vi "Run.vi"(7 "Team Index":i32, 8 "Column":i32, 9 "Row":i32, 10 "View":i32[](array[numeric]) caption="View (Team Index, -1: empty)", 11 "Runner in":refnum<class "Pinwheel.lvclass">) -> (0 "Replicated":refnum<class "Square.lvclass">, 1 "Direction":T1, 2 "Action":T2, 3 "Square Out":refnum<class "Square.lvclass">)   [LabVIEW 2015, in "Pinwheel.lvclass"]
uses:
  Pinwheel.lvclass
  Square/Square.lvclass
  Type Defs/Action Enum.ctl
  Type Defs/Direction Enum.ctl
  DVR Cluster.ctl
  Pinwheel.lvclass/Pinwheel.ctl
  SubVIs/Read-Only Globals.vi
  SubVIs/Globals (private).vi
  Type Defs/SB Type Defs.lvlib
panel:
  # "NW\nN\nNE\nE\nSE\nS\nSW\nW"
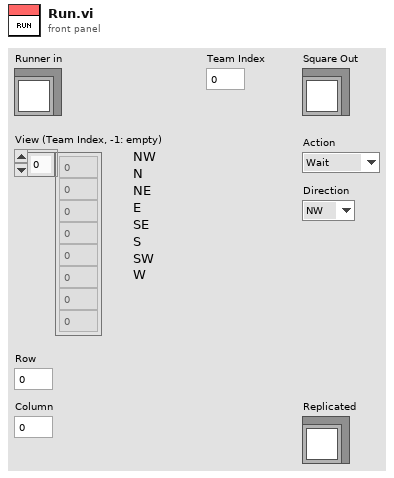
[diagram p1: front panel]
types:
  T1 = typedef "SB Type Defs.lvlib/Direction Enum.ctl" = enum16{"NW", "N", "NE", "E", "SE", "S", "SW", "W"}
  T2 = typedef "SB Type Defs.lvlib/Action Enum.ctl" = enum16{"Wait", "Move", "Attack", "Replicate"}
  T3 = typedef "Pinwheel.lvclass/DVR Cluster.ctl" = cluster{"N":i32, "E":i32, "S":i32, "W":i32, "OD":T1, "NR":i32, "ER":i32, "SR":i32, "WR":i32, "NE":i32, "EE":i32, "SE":i32, "WE":i32, "Team":i32}
  T4 = typedef "Pinwheel.lvclass/Ring Enum.ctl" = enum16{"Defense", "Fill", "Outer", "Inner"}
  T5 = typedef "Pinwheel.lvclass/Role Enum.ctl" = enum16{"Parent", "Move", "Child"}
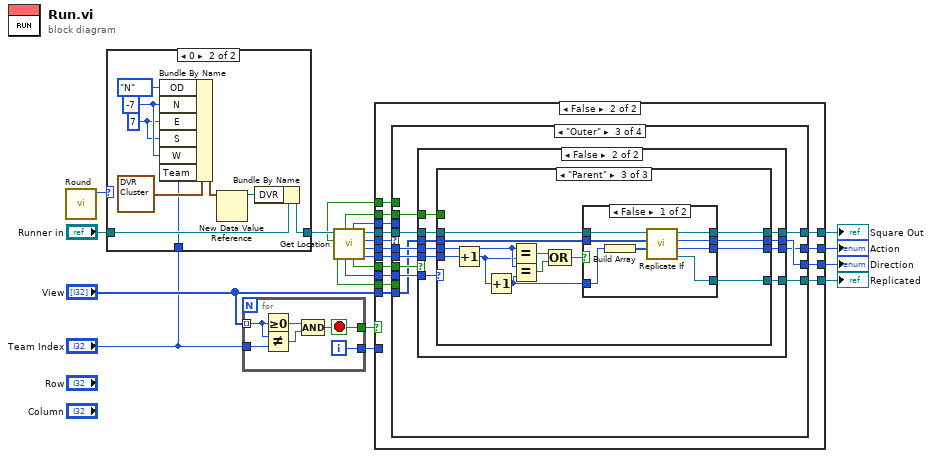
[diagram p0: block diagram]
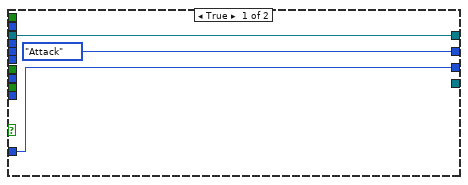
[diagram p2: hidden frame]
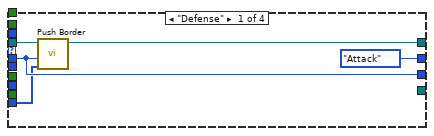
[diagram p3: hidden frame]
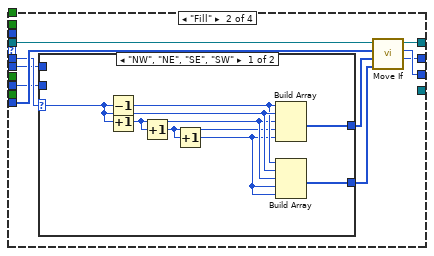
[diagram p4: hidden frame]
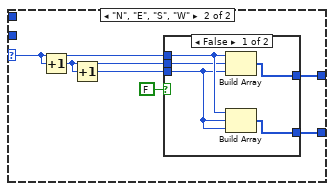
[diagram p5: hidden frame]
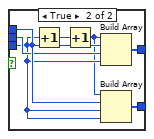
[diagram p6: hidden frame]
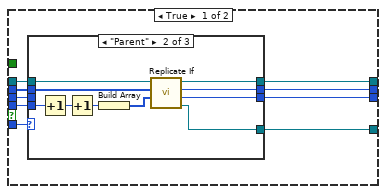
[diagram p7: hidden frame]
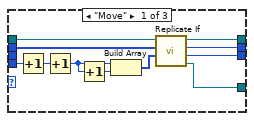
[diagram p8: hidden frame]
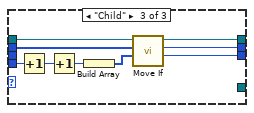
[diagram p9: hidden frame]
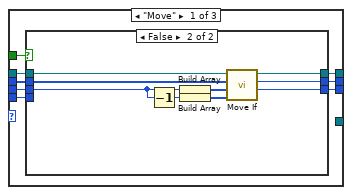
[diagram p10: hidden frame]
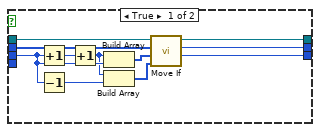
[diagram p11: hidden frame]
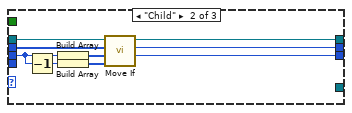
[diagram p12: hidden frame]
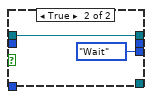
[diagram p13: hidden frame]
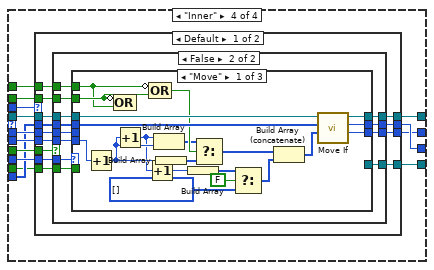
[diagram p14: hidden frame]
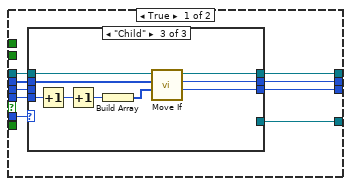
[diagram p15: hidden frame]
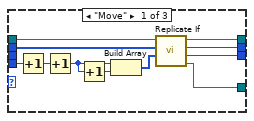
[diagram p16: hidden frame]
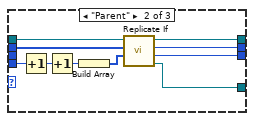
[diagram p17: hidden frame]
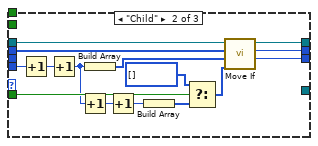
[diagram p18: hidden frame]
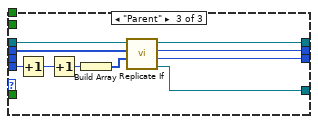
[diagram p19: hidden frame]
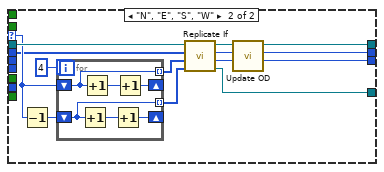
[diagram p20: hidden frame]
diagram:
  n1 = call "Round.vi"() -> ("Round"=w21:i32)  [unwired: 11 in]
  n2 = case shown="0" w21 {
    tunnel: "Runner in" -> [w22 w31]
    tunnel: [w22 w29] -> w19
    tunnel: "Team Index" -> [_ w23]
    frame Default {
    }
    frame 0 {
      w25 = 7 ("E")
      w26 = -7 ("N")
      n3 = Bundle By Name(cluster=T3 {"N"=0, "E"=0, "S"=0, "W"=0, "OD"=enum."NW", "NR"=0, "ER"=0, "SR"=0, "WR"=0, "NE"=0, "EE"=0, "SE"=0, "WE"=0, "Team"=0} ("DVR Cluster"), "OD"=Direction_Enum."N", "N"=w26, "E"=w25, "S"=w25, "W"=w26, "Team"=w23) -> (w27:T3)
      n4 = New Data Value Reference(data value=w27) -> (data value reference=w30:refnum<data-value>)  [unwired: 1 in, 1 out]
      n5 = Bundle By Name(cluster=w31, "DVR"=w30) -> (w29:refnum<class "Pinwheel.lvclass">)
    }
  }
  n6 = for {
    tunnel: "View" -> [w35] mode=indexing
    tunnel: "Team Index" -> [w36]
    tunnel: [w33] -> w3
    tunnel: [w32] -> w2
    i -> [w33]
    stop <- w32 stop-if-true
    n7 = Greater Or Equal To 0?(x=w35) -> (x >= 0?=w37:bool)
    n8 = Not Equal?(x=w35, y=w36) -> (x != y?=w34:bool)
    n9 = Compound Arithmetic op=AND(w37, w34) -> (w32:bool)
  }
  n10 = call "Get Location.vi"("Class"=w19) -> ("Clan"=w11:T1, "Post"=w12:T1, "Ring"=w13:T4, "Class"=w14:refnum<class "Pinwheel.lvclass">, "Diagonal"=w10:bool, "OD"=w8:T1, "Role"=w9:T5, "Jump"=w7:bool, "Move Anyway"=w6:bool, "Chute"=w5:bool)  [unwired: 1 in]
  n11 = case shown="False" w2 {
    tunnel: w14 -> [w40 w55]
    tunnel: [w40 w54] -> w18
    tunnel: [w38 w53] -> w17
    tunnel: [Action_Enum."Attack" ("Action") w52] -> w16
    tunnel: [_ w51] -> w15
    tunnel: "View" -> [_ w50]
    tunnel: w13 -> [_ w49]
    tunnel: w12 -> [_ w48]
    tunnel: w11 -> [_ w47]
    tunnel: w10 -> [_ w46]
    tunnel: w9 -> [_ w45]
    tunnel: w8 -> [_ w44]
    tunnel: w7 -> [_ w43]
    tunnel: w6 -> [_ w42]
    tunnel: w5 -> [_ w41]
    tunnel: w3 -> [w38 _]
    frame True {
    }
    frame False {
      n12 = case shown="\"Outer\"" w49 {
        tunnel: [w58 w69 w101 w224] -> w54
        tunnel: w55 -> [w59 w70 w102 w225]
        tunnel: w48 -> [w57 w65 w104 w227]
        tunnel: w50 -> [w56 w68 w98 w221]
        tunnel: [w57 w67 w100 w223] -> w53
        tunnel: [Action_Enum."Attack" ("Action") w66 w99 w222] -> w52
        tunnel: [_ _ w97 w220] -> w51
        tunnel: w47 -> [_ w61 w103 w226]
        tunnel: w46 -> [_ _ w106 w229]
        tunnel: w45 -> [_ w62 w105 w228]
        tunnel: w44 -> [_ _ _ w219]
        tunnel: w43 -> [_ _ w96 w218]
        tunnel: w42 -> [_ _ _ w217]
        tunnel: w41 -> [_ _ _ w216]
        frame "Defense" {
          n13 = call "Push Border.vi"("1D Maze"=w56, "Post"=w57, "Class"=w59) -> ("Class"=w58:refnum<class "Pinwheel.lvclass">)  [unwired: 8 in]
        }
        frame "Fill" {
          n14 = case shown="\"NW\", \"NE\", \"SE\", \"SW\"" w65 {
            selector: w65 -> [w77 w83]
            tunnel: [w76 w82] -> w64
            tunnel: [w75 w81] -> w63
            tunnel: w62 -> [_ _]
            tunnel: w61 -> [_ _]
            frame "NW", "NE", "SE", "SW" {
              n15 = Decrement(x=w77) -> (x-1=w74:T1)
              n16 = Increment(x=w77) -> (x+1=w73:T1)
              n17 = Increment(x=w73) -> (x+1=w72:T1)
              n18 = Increment(x=w72) -> (x+1=w71:T1)
              n19 = Build Array(w74, w77, w73, w72, w71) -> (w76:T1[])
              n20 = Build Array(w74, w77, w73, w71, w71) -> (w75:T1[])
            }
            frame "N", "E", "S", "W" {
              n21 = Increment(x=w83) -> (x+1=w80:T1)
              n22 = Increment(x=w80) -> (x+1=w79:T1)
              n23 = case shown="False" FALSE {
                tunnel: [w88 w95] -> w82
                tunnel: w83 -> [w87 w94]
                tunnel: w80 -> [w86 w93]
                tunnel: [w85 w92] -> w81
                tunnel: w79 -> [w84 w91]
                frame False {
                  n24 = Build Array(w87, w86, w84) -> (w88:T1[])
                  n25 = Build Array(w87, w84, w84) -> (w85:T1[])
                }
                frame True {
                  n26 = Increment(x=w91) -> (x+1=w90:T1)
                  n27 = Increment(x=w90) -> (x+1=w89:T1)
                  n28 = Build Array(w89, w94, w93, w91) -> (w95:T1[])
                  n29 = Build Array(w89, w94, w91, w91) -> (w92:T1[])
                }
              }
            }
          }
          n30 = call "Move If.vi"("If"=w63, "Move"=w64, "1D Maze"=w68, "Class"=w70) -> ("Action"=w66:T2, "Direction"=w67:T1, "Class"=w69:refnum<class "Pinwheel.lvclass">)  [unwired: 5 in]
        }
        frame "Outer" {
          n31 = case shown="False" w106 {
            tunnel: w105 -> [w115 w155]
            tunnel: w104 -> [w114 w154]
            tunnel: w103 -> [w113 w153]
            tunnel: w102 -> [w112 w152]
            tunnel: [w111 w151] -> w101
            tunnel: [w110 w150] -> w100
            tunnel: [w109 w149] -> w99
            tunnel: w98 -> [w108 w148]
            tunnel: [w107 w147] -> w97
            tunnel: w96 -> [_ w146]
            frame True {
              n32 = case shown="\"Parent\"" w115 {
                tunnel: w114 -> [_ _ _]
                tunnel: w113 -> [w124 w130 w145]
                tunnel: w112 -> [w126 w136 w142]
                tunnel: [w118 w131 w141] -> w111
                tunnel: [w119 w132 w140] -> w110
                tunnel: [w120 w133 w139] -> w109
                tunnel: w108 -> [w125 w135 w138]
                tunnel: [w121 w134 _] -> w107
                frame "Move" {
                  n33 = Increment(x=w124) -> (x+1=w123:T1)
                  n34 = Increment(x=w123) -> (x+1=w116:T1)
                  n35 = Increment(x=w116) -> (x+1=w117:T1)
                  n36 = Build Array(w116, w117) -> (w122:T1[])
                  n37 = call "Replicate If.vi"("Replicate"=w122, "1D Maze"=w125, "Class"=w126) -> ("Replicated"=w121:refnum<class "Pinwheel.lvclass">, "Action"=w120:T2, "Direction"=w119:T1, "Class"=w118:refnum<class "Pinwheel.lvclass">)  [unwired: 5 in]
                }
                frame "Parent" {
                  n38 = Increment(x=w130) -> (x+1=w127:T1)
                  n39 = Increment(x=w127) -> (x+1=w128:T1)
                  n40 = Build Array(w128) -> (w129:T1[])
                  n41 = call "Replicate If.vi"("Replicate"=w129, "1D Maze"=w135, "Class"=w136) -> ("Replicated"=w134:refnum<class "Pinwheel.lvclass">, "Action"=w133:T2, "Direction"=w132:T1, "Class"=w131:refnum<class "Pinwheel.lvclass">)  [unwired: 5 in]
                }
                frame "Child" {
                  n42 = Increment(x=w145) -> (x+1=w144:T1)
                  n43 = Increment(x=w144) -> (x+1=w143:T1)
                  n44 = Build Array(w143) -> (w137:T1[])
                  n45 = call "Move If.vi"("Move"=w137, "1D Maze"=w138, "Class"=w142) -> ("Action"=w139:T2, "Direction"=w140:T1, "Class"=w141:refnum<class "Pinwheel.lvclass">)  [unwired: 6 in]
                }
              }
            }
            frame False {
              n46 = case shown="\"Parent\"" w155 {
                tunnel: w154 -> [w158 w184 w198]
                tunnel: w153 -> [w156 _ w199]
                tunnel: w152 -> [w163 w192 w205]
                tunnel: [w162 w191 w200] -> w151
                tunnel: [w161 w190 w201] -> w150
                tunnel: [w160 w189 w202] -> w149
                tunnel: w148 -> [w159 w188 w204]
                tunnel: [_ _ w203] -> w147
                tunnel: w146 -> [w157 _ _]
                frame "Move" {
                  n47 = case shown="False" w157 {
                    tunnel: w163 -> [w174 w183]
                    tunnel: [w164 w182] -> w162
                    tunnel: [w166 w181] -> w161
                    tunnel: [w173 w180] -> w160
                    tunnel: w159 -> [w172 w179]
                    tunnel: w158 -> [w169 w178]
                    tunnel: w156 -> [_ _]
                    frame True {
                      n48 = Increment(x=w169) -> (x+1=w165:T1)
                      n49 = Decrement(x=w169) -> (x-1=w168:T1)
                      n50 = Increment(x=w165) -> (x+1=w167:T1)
                      n51 = Build Array(w167, w169) -> (w171:T1[])
                      n52 = Build Array(w167, w168) -> (w170:T1[])
                      n53 = call "Move If.vi"("If"=w170, "Move"=w171, "1D Maze"=w172, "Class"=w174) -> ("Action"=w173:T2, "Direction"=w166:T1, "Class"=w164:refnum<class "Pinwheel.lvclass">)  [unwired: 5 in]
                    }
                    frame False {
                      n54 = Decrement(x=w178) -> (x-1=w176:T1)
                      n55 = Build Array(w178) -> (w177:T1[])
                      n56 = Build Array(w176) -> (w175:T1[])
                      n57 = call "Move If.vi"("If"=w175, "Move"=w177, "1D Maze"=w179, "Class"=w183) -> ("Action"=w180:T2, "Direction"=w181:T1, "Class"=w182:refnum<class "Pinwheel.lvclass">)  [unwired: 5 in]
                    }
                  }
                }
                frame "Child" {
                  n58 = Decrement(x=w184) -> (x-1=w186:T1)
                  n59 = Build Array(w184) -> (w187:T1[])
                  n60 = Build Array(w186) -> (w185:T1[])
                  n61 = call "Move If.vi"("If"=w185, "Move"=w187, "1D Maze"=w188, "Class"=w192) -> ("Action"=w189:T2, "Direction"=w190:T1, "Class"=w191:refnum<class "Pinwheel.lvclass">)  [unwired: 5 in]
                }
                frame "Parent" {
                  n62 = Increment(x=w199) -> (x+1=w197:T1)
                  n63 = Increment(x=w197) -> (x+1=w193:T1)
                  n64 = Equal?(x=w198, y=w197) -> (x = y?=w196:bool)
                  n65 = Equal?(x=w198, y=w193) -> (x = y?=w195:bool)
                  n66 = Compound Arithmetic op=OR(w196, w195) -> (w194:bool)
                  n67 = case shown="False" w194 {
                    tunnel: w205 -> [w213 w215]
                    tunnel: w204 -> [w212 _]
                    tunnel: [w210 _] -> w203
                    tunnel: [w209 Action_Enum."Wait" ("Action")] -> w202
                    tunnel: [w208 _] -> w201
                    tunnel: [w207 w215] -> w200
                    tunnel: w193 -> [w206 _]
                    frame False {
                      n68 = Build Array(w206) -> (w211:T1[])
                      n69 = call "Replicate If.vi"("Replicate"=w211, "1D Maze"=w212, "Class"=w213) -> ("Replicated"=w210:refnum<class "Pinwheel.lvclass">, "Action"=w209:T2, "Direction"=w208:T1, "Class"=w207:refnum<class "Pinwheel.lvclass">)  [unwired: 5 in]
                    }
                    frame True {
                    }
                  }
                }
              }
            }
          }
        }
        frame "Inner" {
          n70 = case shown="Default" w219 {
            selector: w219 -> [_ w348]
            tunnel: w229 -> [w242 _]
            tunnel: w228 -> [w241 _]
            tunnel: w227 -> [w240 _]
            tunnel: w226 -> [w239 _]
            tunnel: w225 -> [w238 w350]
            tunnel: [w237 w342] -> w224
            tunnel: [w236 w339] -> w223
            tunnel: [w235 w341] -> w222
            tunnel: w221 -> [w234 w347]
            tunnel: [w233 w340] -> w220
            tunnel: w218 -> [w232 _]
            tunnel: w217 -> [w231 _]
            tunnel: w216 -> [w230 _]
            frame Default {
              n71 = case shown="False" w242 {
                tunnel: w241 -> [w251 w293]
                tunnel: w240 -> [w250 w292]
                tunnel: w239 -> [w249 w291]
                tunnel: w238 -> [w248 w290]
                tunnel: [w247 w289] -> w237
                tunnel: [w246 w288] -> w236
                tunnel: [w245 w287] -> w235
                tunnel: w234 -> [w244 w286]
                tunnel: [w243 w285] -> w233
                tunnel: w232 -> [_ w283]
                tunnel: w231 -> [_ w284]
                tunnel: w230 -> [_ w282]
                frame True {
                  n72 = case shown="\"Child\"" w251 {
                    tunnel: w250 -> [_ _ _]
                    tunnel: w249 -> [w260 w266 w281]
                    tunnel: w248 -> [w262 w272 w278]
                    tunnel: [w254 w267 w277] -> w247
                    tunnel: [w255 w268 w276] -> w246
                    tunnel: [w256 w269 w275] -> w245
                    tunnel: w244 -> [w261 w271 w274]
                    tunnel: [w257 w270 _] -> w243
                    frame "Move" {
                      n73 = Increment(x=w260) -> (x+1=w259:T1)
                      n74 = Increment(x=w259) -> (x+1=w252:T1)
                      n75 = Increment(x=w252) -> (x+1=w253:T1)
                      n76 = Build Array(w252, w253) -> (w258:T1[])
                      n77 = call "Replicate If.vi"("Replicate"=w258, "1D Maze"=w261, "Class"=w262) -> ("Replicated"=w257:refnum<class "Pinwheel.lvclass">, "Action"=w256:T2, "Direction"=w255:T1, "Class"=w254:refnum<class "Pinwheel.lvclass">)  [unwired: 5 in]
                    }
                    frame "Parent" {
                      n78 = Increment(x=w266) -> (x+1=w263:T1)
                      n79 = Increment(x=w263) -> (x+1=w264:T1)
                      n80 = Build Array(w264) -> (w265:T1[])
                      n81 = call "Replicate If.vi"("Replicate"=w265, "1D Maze"=w271, "Class"=w272) -> ("Replicated"=w270:refnum<class "Pinwheel.lvclass">, "Action"=w269:T2, "Direction"=w268:T1, "Class"=w267:refnum<class "Pinwheel.lvclass">)  [unwired: 5 in]
                    }
                    frame "Child" {
                      n82 = Increment(x=w281) -> (x+1=w280:T1)
                      n83 = Increment(x=w280) -> (x+1=w279:T1)
                      n84 = Build Array(w279) -> (w273:T1[])
                      n85 = call "Move If.vi"("Move"=w273, "1D Maze"=w274, "Class"=w278) -> ("Action"=w275:T2, "Direction"=w276:T1, "Class"=w277:refnum<class "Pinwheel.lvclass">)  [unwired: 6 in]
                    }
                  }
                }
                frame False {
                  n86 = case shown="\"Move\"" w293 {
                    tunnel: w292 -> [_ _ _]
                    tunnel: w291 -> [w306 w323 w332]
                    tunnel: w290 -> [w313 w328 w338]
                    tunnel: [w304 w327 w333] -> w289
                    tunnel: [w311 w326 w334] -> w288
                    tunnel: [w305 w325 w335] -> w287
                    tunnel: w286 -> [w312 w324 w337]
                    tunnel: [_ _ w336] -> w285
                    tunnel: w284 -> [_ w320 _]
                    tunnel: w283 -> [w303 _ _]
                    tunnel: w282 -> [w302 _ _]
                    frame "Move" {
                      w299 = T1[] [] items=["NW", "N", "NE", "E", "SE", "S", "SW", "W"] ("s? t:f")
                      n87 = Increment(x=w306) -> (x+1=w310:T1)
                      n88 = Compound Arithmetic op=OR(invert w303, w302) -> ()  [unwired: 1 out]
                      n89 = Increment(x=w310) -> (x+1=w297:T1)
                      n90 = Increment(x=w297) -> (x+1=w296:T1)
                      n91 = Compound Arithmetic op=OR(invert w302, w303) -> (w309:bool)
                      n92 = Build Array(w297, w310) -> (w308:T1[])
                      n93 = Build Array(w310) -> (w307:T1[])
                      n94 = Build Array(w296) -> (w295:T1[])
                      n95 = Select(t=w308, s=w309, f=w307) -> (s? t:f=w301:T1[])
                      n96 = Select(t=w295, s=FALSE, f=w299) -> (s? t:f=w298:T1[])
                      n97 = Build Array (concatenate)(w301, w298) -> (w300:T1[])
                      n98 = call "Move If.vi"("Move"=w300, "1D Maze"=w312, "Class"=w313) -> ("Action"=w305:T2, "Direction"=w311:T1, "Class"=w304:refnum<class "Pinwheel.lvclass">)  [unwired: 6 in]
                    }
                    frame "Child" {
                      w314 = T1[] [] items=["NW", "N", "NE", "E", "SE", "S", "SW", "W"] ("t")
                      n99 = Increment(x=w323) -> (x+1=w322:T1)
                      n100 = Increment(x=w322) -> (x+1=w317:T1)
                      n101 = Increment(x=w317) -> (x+1=w318:T1)
                      n102 = Build Array(w317) -> (w321:T1[])
                      n103 = Increment(x=w318) -> (x+1=w319:T1)
                      n104 = Build Array(w319) -> (w316:T1[])
                      n105 = Select(t=w314, s=w320, f=w316) -> (s? t:f=w315:T1[])
                      n106 = call "Move If.vi"("If"=w315, "Move"=w321, "1D Maze"=w324, "Class"=w328) -> ("Action"=w325:T2, "Direction"=w326:T1, "Class"=w327:refnum<class "Pinwheel.lvclass">)  [unwired: 5 in]
                    }
                    frame "Parent" {
                      n107 = Increment(x=w332) -> (x+1=w329:T1)
                      n108 = Increment(x=w329) -> (x+1=w331:T1)
                      n109 = Build Array(w331) -> (w330:T1[])
                      n110 = call "Replicate If.vi"("Replicate"=w330, "1D Maze"=w337, "Class"=w338) -> ("Replicated"=w336:refnum<class "Pinwheel.lvclass">, "Action"=w335:T2, "Direction"=w334:T1, "Class"=w333:refnum<class "Pinwheel.lvclass">)  [unwired: 5 in]
                    }
                  }
                }
              }
            }
            frame "N", "E", "S", "W" {
              n111 = Decrement(x=w348) -> (x-1=w345:T1)
              n112 = for {
                N: 4 -> [_]
                shift-right: [w354] -> _
                shift-left: w348 -> [w356]
                tunnel: [w356] -> w346 mode=indexing
                shift-right: [w352] -> _
                shift-left: w345 -> [w351]
                tunnel: [w351] -> w344 mode=indexing
                n113 = Increment(x=w351) -> (x+1=w353:T1)
                n114 = Increment(x=w356) -> (x+1=w355:T1)
                n115 = Increment(x=w353) -> (x+1=w352:T1)
                n116 = Increment(x=w355) -> (x+1=w354:T1)
              }
              n117 = call "Replicate If.vi"("If"=w344, "Replicate"=w346, "1D Maze"=w347, "Class"=w350) -> ("Replicated"=w340:refnum<class "Pinwheel.lvclass">, "Action"=w341:T2, "Direction"=w339:T1, "Class"=w343:refnum<class "Pinwheel.lvclass">)  [unwired: 4 in]
              n118 = call "Update OD.vi"("Action"=w341, "Direction"=w339, "Class"=w343) -> ("Class"=w342:refnum<class "Pinwheel.lvclass">)  [unwired: 8 in]
            }
          }
        }
      }
    }
  }
  "Square Out" <- w18
  "Action" <- w16
  "Direction" <- w17
  "Replicated" <- w15
